vi "PH_Beckhoff_PP_PU.set i Attr and start DIM Services for Trigger.vi"(3 "error in":errorcluster, 4 "Values":T4, 5 "PU Type":T3=enum."PA 19mm") -> (0 "error out":errorcluster, 1 "Trigger":T2(array[cluster]) {"Status"."Status" items=["no info", "off/false/out", "on/true/in", "Failure", "Alarm", "Status 1", "Status 2", "Status 3"]})   [LabVIEW 2014, in "PH_Beckhoff_PP_PU.lvlib"]
uses:
  PH_Beckhoff_PP_PU.lvlib
  PH_Beckhoff/PH_Beckhoff.Values.ctl
  PH_Beckhoff/PH_Beckhoff.Sonderklemmen Inputs.ctl
  PH_Beckhoff/PH_Beckhoff.Analog Inputs.ctl
  PH_Beckhoff/PH_Beckhoff.Scaling Type.ctl
  PH_Beckhoff/PH_Beckhoff.Analog Outputs.ctl
  PH_Beckhoff/PH_Beckhoff.Digital Inputs.ctl
  PH_Beckhoff/PH_Beckhoff.Digital Outputs.ctl
  PH_Beckhoff_PP_PU.PU Rack Type.ctl
  PH_Basics/PH_StatusHandler/PH_StatusHandler.Status.ctl
  PH_Basics/PH_PP_Common/PH_PP_Common.Trigger Tags.ctl
  CSlibraries-extern/DimLVEvent/LVDimInterface/LVDimInterface.lvlib
  PH_Basics/PH_StatusHandler/PH_StatusHandler.lvlib
  CSlibraries/UtilityLib/UtilityLib.lvlib
  PH_Basics/PH_PP_Common/PH_PP_Common.lvlib
  PH_Beckhoff/PH_Beckhoff.lvlib
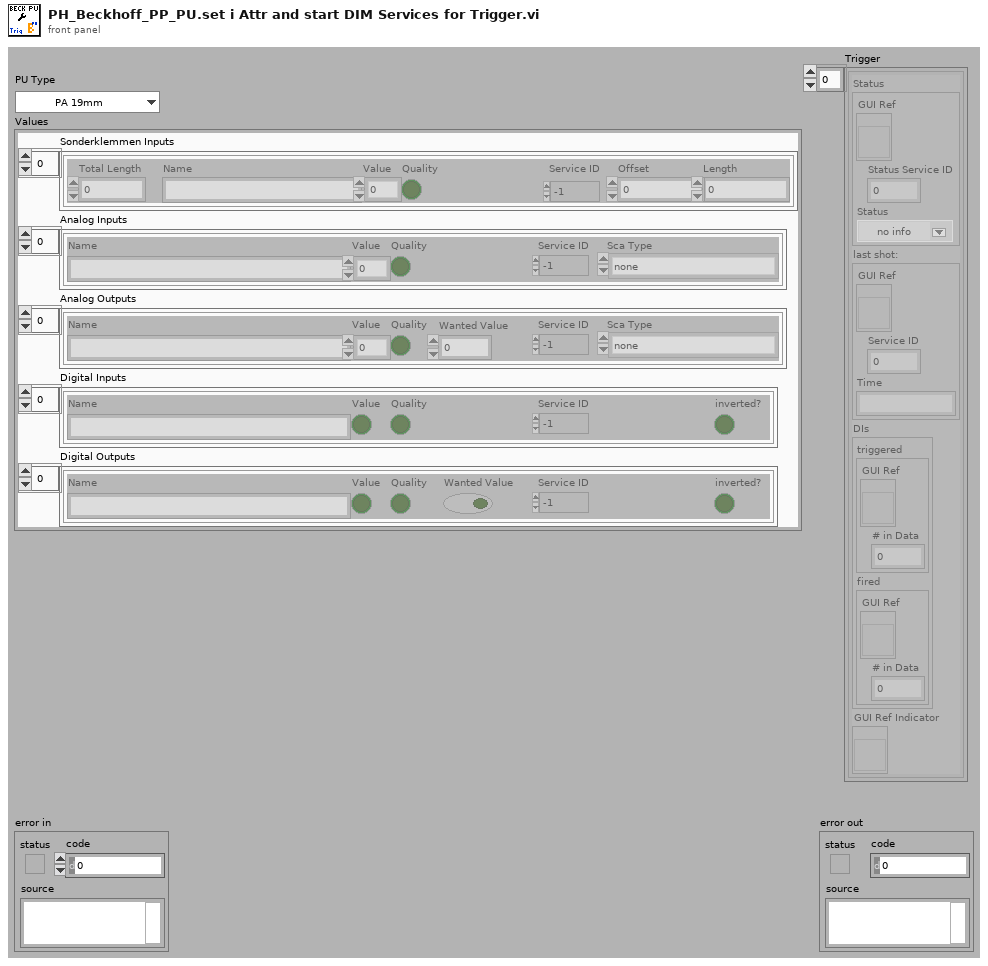
[diagram p1: front panel]
types:
  T1 = typedef "PH_StatusHandler.lvlib/PH_StatusHandler.Status.ctl" = i16
  T2 = cluster{"Status":cluster{"GUI Ref":refnum<vi>, "Status Service ID":i32, "Status":T1}, "last shot:":cluster{"GUI Ref":refnum<vi>, "Service ID":i32, "Time":string}, "DIs":cluster{"triggered":cluster{"GUI Ref":refnum<vi>, "# in Data":i32}, "fired":cluster{"GUI Ref":refnum<vi>, "# in Data":i32}}, "GUI Ref Indicator":refnum<vi>}[]
  T3 = typedef "PH_Beckhoff_PP_PU.lvlib/PH_Beckhoff_PP_PU.PU Rack Type.ctl" = enum16{"no Info", "PA 19mm", "PA 45mm", "MA PU 1 and 2", "MA PU 3 and 4", "MA PU 5 and 6", "MA FR and PILC"}
  T4 = typedef "PH_Beckhoff.lvlib/PH_Beckhoff.Values.ctl" = cluster{"Sonderklemmen Inputs":T5, "Analog Inputs":T6, "Analog Outputs":T8, "Digital Inputs":T9, "Digital Outputs":T10}
  T5 = typedef "PH_Beckhoff.lvlib/PH_Beckhoff.Sonderklemmen Inputs.ctl" = cluster{"Total Length":u32, "Name":string, "Value":u64, "Quality":bool, "Service ID":i32, "Offset":u32, "Length":u32}[]
  T6 = typedef "PH_Beckhoff.lvlib/PH_Beckhoff.Analog Inputs.ctl" = cluster{"Name":string, "Value":u32, "Quality":bool, "Service ID":i32, "Sca Type":T7}[]
  T7 = typedef "PH_Beckhoff.lvlib/PH_Beckhoff.Scaling Type.ctl" = enum16{"none", "0 ... 15 Bit -> 0 ... 5", "0 ... 15 Bit -> 0 ... 10", "0 ... 15 Bit -> 0 ... 25", "0 ... 15 Bit -> 4 ... 20", "0 ... 15 Bit -> 0 ... 1", "0 ... 15 Bit -> 0 ... 20000", "0 ... 15 Bit -> 0 ... 24000"}
  T8 = typedef "PH_Beckhoff.lvlib/PH_Beckhoff.Analog Outputs.ctl" = cluster{"Name":string, "Value":u32, "Quality":bool, "Wanted Value":u32, "Service ID":i32, "Sca Type":T7}[]
  T9 = typedef "PH_Beckhoff.lvlib/PH_Beckhoff.Digital Inputs.ctl" = cluster{"Name":string, "Value":bool, "Quality":bool, "Service ID":i32, "inverted?":bool}[]
  T10 = typedef "PH_Beckhoff.lvlib/PH_Beckhoff.Digital Outputs.ctl" = cluster{"Name":string, "Value":bool, "Quality":bool, "Wanted Value":bool, "Service ID":i32, "inverted?":bool}[]
  T11 = typedef "PH_PP_Common.lvlib/PH_PP_Common.Trigger Tags.ctl" = enum16{"triggered", "fired", "Status", "Last Shot"}
  T12 = typedef "PH_PP_Common.lvlib/PH_PP_Common.PUs.ctl" = enum16{"no Info", "PA-19mm-1", "PA-19mm-2", "PA-45mm-PILC", "PA-45mm-MAIN", "MA-PU-1", "MA-PU-2", "MA-PU-3", "MA-PU-4", "MA-PU-5", "MA-PU-6", "MA-FR", "MA-PILC", "PA-45mm-DP"}
  T13 = cluster{"Status":cluster{"GUI Ref":refnum<vi>, "Status Service ID":i32, "Status":T1}, "last shot:":cluster{"GUI Ref":refnum<vi>, "Service ID":i32, "Time":string}, "DIs":cluster{"triggered":cluster{"GUI Ref":refnum<vi>, "# in Data":i32}, "fired":cluster{"GUI Ref":refnum<vi>, "# in Data":i32}}, "GUI Ref Indicator":refnum<vi>}
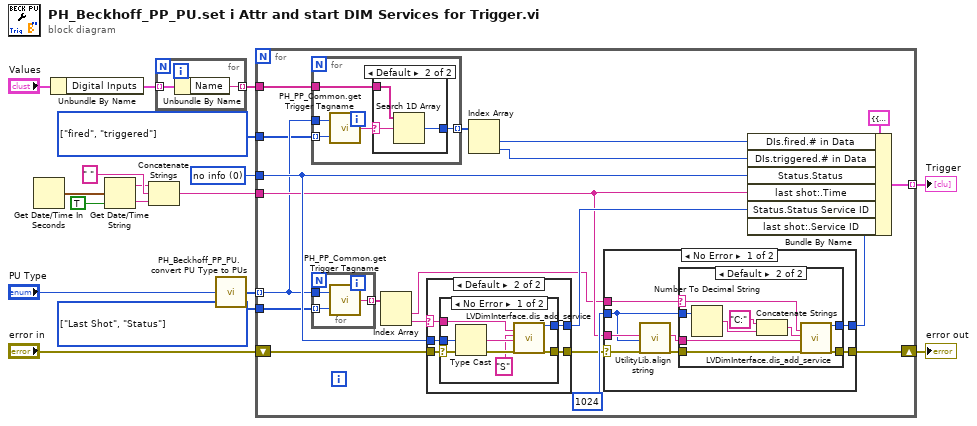
[diagram p0: block diagram]
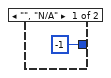
[diagram p2: hidden frame]
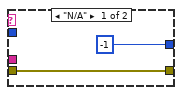
[diagram p3: hidden frame]
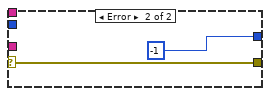
[diagram p4: hidden frame]
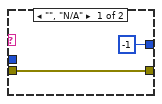
[diagram p5: hidden frame]
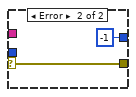
[diagram p6: hidden frame]
diagram:
  w6 = T11[] [enum."fired", enum."triggered"] items=["triggered", "fired", "Status", "Last Shot"]
  w9 = T11[] [enum."Last Shot", enum."Status"] items=["triggered", "fired", "Status", "Last Shot"]
  w15 = T1 0 items=["no info", "off/false/out", "on/true/in", "Failure", "Alarm", "Status 1", "Status 2", "Status 3"] ("Status")
  n1 = Get Date/Time In Seconds() -> (seconds since 1Jan1904=w12:timestamp)
  n2 = Unbundle By Name("Values") -> ("Digital Inputs"=w4:T9)
  n3 = Get Date/Time String(seconds (now)=w12, want seconds? (F)=TRUE) -> (date string=w11:string, time string=w10:string)  [unwired: 1 in]
  n4 = Concatenate Strings(w11, " " ("string"), w10) -> (w8:string)
  n5 = for {
    tunnel: w4 -> [w19] mode=indexing
    tunnel: [w18] -> w5 mode=indexing
    n6 = Unbundle By Name(w19) -> ("Name"=w18:string)
  }
  n7 = call "PH_Beckhoff_PP_PU.convert PU Type to PUs.vi"("PU Type"="PU Type") -> ("PUs"=w14:T12[])
  n8 = for {
    shift-right: [w32] -> w2
    shift-left: "error in" -> [w36]
    tunnel: [w39] -> w1 mode=indexing
    tunnel: w15 -> [w38]
    tunnel: w14 -> [w25] mode=indexing
    tunnel: w9 -> [w27]
    tunnel: w8 -> [w29]
    tunnel: w6 -> [w24]
    tunnel: w5 -> [w23]
    n9 = for {
      tunnel: w25 -> [w44]
      tunnel: w24 -> [w43] mode=indexing
      tunnel: [w40] -> w26 mode=indexing
      tunnel: w23 -> [w41]
      n10 = call "PH_PP_Common.get Trigger Tagname.vi"("Trigger Tag"=w43, "PU"=w44) -> ("Trigger Tagname"=w42:string)
      n11 = case shown="Default" w42 {
        selector: w42 -> [_ w48]
        tunnel: w41 -> [_ w47]
        tunnel: [-1 ("index of element") w46] -> w40
        frame "", "N/A" {
        }
        frame Default {
          n12 = Search 1D Array(1D array=w47, element=w48) -> (index of element=w46:i32)  [unwired: 1 in]
        }
      }
    }
    n13 = for {
      tunnel: w25 -> [w72]
      tunnel: w27 -> [w70] mode=indexing
      tunnel: [w71] -> w35 mode=indexing
      n14 = call "PH_PP_Common.get Trigger Tagname.vi"("Trigger Tag"=w70, "PU"=w72) -> ("Trigger Tagname"=w71:string)
    }
    n15 = Index Array(array=w35) -> (element #1=w28:string, element #2=w34:string)  [unwired: 2 in]
    n16 = case shown="Default" w34 {
      selector: w34 -> [_ w75]
      tunnel: w36 -> [w74 w79]
      tunnel: [w74 w78] -> w31
      tunnel: [-1 ("my_serviceID") w77] -> w37
      tunnel: w38 -> [_ w76]
      frame "", "N/A" {
      }
      frame Default {
        n17 = case shown="No Error" w79 {
          selector: w79 -> [w84 w88]
          tunnel: [w86 -1 ("my_serviceID")] -> w77
          tunnel: [w85 w88] -> w78
          tunnel: w76 -> [w83 _]
          tunnel: w75 -> [w80 _]
          frame No Error {
            n18 = Type Cast(x=w83) -> (*(type *) &x=w82:string)  [unwired: 1 in]
            n19 = call "LVDimInterface.dis_add_service.vi"("serviceName"=w80, "typeDescriptor"="S", "data"=w82, "error in (no error)"=w84) -> ("my_serviceID"=w86:i32, "error out"=w85:errorcluster)  [unwired: 14 in]
          }
          frame Error {
          }
        }
      }
    }
    n20 = Index Array(array=w26) -> (element #1=w21:i32, element #2=w22:i32)  [unwired: 2 in]
    n21 = case shown="No Error" w31 {
      selector: w31 -> [w49 w69]
      tunnel: [w56 -1 ("my_serviceID")] -> w30
      tunnel: [w55 w69] -> w32
      tunnel: w29 -> [w54 _]
      tunnel: w28 -> [w53 _]
      tunnel: u16 1024 ("String Length (1024)") -> [w50 _]
      frame No Error {
        n22 = call "UtilityLib.align string.vi"("stringIn"=w54, "stringLength (80)"=w50, "error in (no error)"=w49) -> ("stringOut"=w52:string, "error out"=w51:errorcluster)  [unwired: 15 in]
        n23 = case shown="Default" w53 {
          selector: w53 -> [_ w59]
          tunnel: [-1 ("my_serviceID") w67] -> w56
          tunnel: [w58 w66] -> w55
          tunnel: w51 -> [w58 w65]
          tunnel: w52 -> [_ w64]
          tunnel: w50 -> [_ w60]
          frame "N/A" {
          }
          frame Default {
            n24 = Number To Decimal String(number=w60) -> (decimal integer string=w61:string)  [unwired: 1 in]
            n25 = Concatenate Strings("C:" ("typeDescriptor"), w61) -> (w62:string)
            n26 = call "LVDimInterface.dis_add_service.vi"("serviceName"=w59, "typeDescriptor"=w62, "data"=w64, "error in (no error)"=w65) -> ("my_serviceID"=w67:i32, "error out"=w66:errorcluster)  [unwired: 14 in]
          }
        }
      }
      frame Error {
      }
    }
    n27 = Bundle By Name(cluster=T13 {"Status"={"GUI Ref"=refnum, "Status Service ID"=0, "Status"=0}, "last shot:"={"GUI Ref"=refnum, "Service ID"=0, "Time"=""}, "DIs"={"triggered"={"GUI Ref"=refnum, "# in Data"=0}, "fired"={"GUI Ref"=refnum, "# in Data"=0}}, "GUI Ref Indicator"=refnum} ("Trigger Data"), "DIs.fired.# in Data"=w21, "DIs.triggered.# in Data"=w22, "Status.Status"=w38, "last shot:.Time"=w29, "Status.Status Service ID"=w37, "last shot:.Service ID"=w30) -> (w39:T13)
  }
  "error out" <- w2
  "Trigger" <- w1
